vi "判决门限数组.vi"(1 "尝试次数":i32=600, 2 "Start":dbl=0.2 format="%#_13g") -> (0 "判决门限数组":dbl[](array[numeric]))   [LabVIEW 2020]
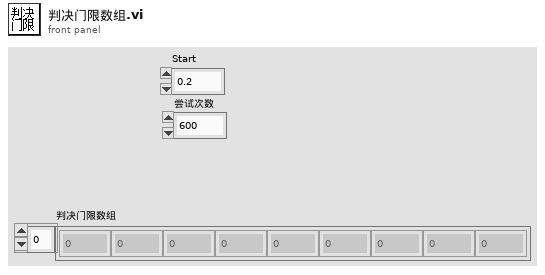
[diagram p1: front panel]
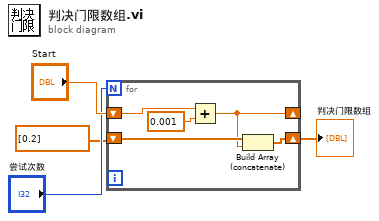
[diagram p0: block diagram]
diagram:
  n1 = for {
    N: "尝试次数" -> [_]
    shift-right: [w5] -> _
    shift-left: "Start" -> [w7]
    shift-right: [w6] -> w2
    shift-left: dbl[] [0.2] -> [w8]
    n2 = Add(x=w7, y=0.001) -> (x+y=w5:dbl)
    n3 = Build Array (concatenate)(w8, w5) -> (w6:dbl[])
  }
  "判决门限数组" <- w2
